vi "Tausand AB1000 Time-Correlated Single Photon Counting Histogram (ContinuousRead) Example.vi"() -> ()   [LabVIEW 2015]
uses:
  <instrlib>/Tausand AB1000/Public/Controls/deviceTypeRing.ctl
  <instrlib>/Tausand AB1000/Public/Controls/channelRing.ctl
  <instrlib>/Tausand AB1000/Public/Controls/settings4ch.ctl
  <instrlib>/Tausand AB1000/Public/Controls/configMultipleCoincRing.ctl
  <vilib>/Utility/error.llb/DialogType.ctl
  <vilib>/Utility/file.llb/Write Delimited Spreadsheet (string).vi
  <vilib>/Analysis/baseanly.llb/Mean (DBL).vi
  <vilib>/Utility/file.llb/Write Delimited Spreadsheet (I64).vi
  <instrlib>/Tausand AB1000/Tausand AB1000.lvlib
  <vilib>/Analysis/NI_AALPro.lvlib
  <vilib>/Analysis/NI_AALBase.lvlib
panel:
  out "read time":timestamp
  out "start time":timestamp
  out "saved headers?":bool
  out "avg data":dbl[][](array[numeric])
  in  "fixed controls":enum32{"Page 1", "Page 2"}(tab)
  in  "Tausand Abacus settings":T1={"sampling"=10, "coincidence_window"=2, "delay_A"=0, "delay_B"=0, "delay_C"=0, "delay_D"=0, "sleep_A"=0, "sleep_B"=0, "sleep_C"=0, "sleep_D"=0, "config_multiple_1"=240} {"config_multiple_1" items=["ABC"=224, "ABD"=208, "ACD"=176, "BCD"=112, "ABCD"=240]; "sleep_D" max=100 step=1; "sleep_C" max=100 step=1; "sleep_B" max=100 step=1; "sleep_A" max=100 step=1; "delay_D" max=100 step=1; "delay_C" max=100 step=1; "delay_B" max=100 step=1; "delay_A" max=100 step=1; "coincidence_window" min=1 max=10000 step=1; "sampling" items=["1ms"=1, "2ms"=2, "3ms"=3, "4ms"=4, "5ms"=5, "6ms"=6, "7ms"=7, "8ms"=8, "9ms"=9, "10ms"=10, "11ms"=11, "12ms"=12, "13ms"=13, "14ms"=14, "15ms"=15, "16ms"=16, "17ms"=17, "18ms"=18, "19ms"=19, "20ms"=20, "21ms"=21, "22ms"=22, "23ms"=23, "24ms"=24, "25ms"=25, "26ms"=26, "27ms"=27, "28ms"=28, "29ms"=29, "30ms"=30, "31ms"=31, "32ms"=32, "33ms"=33, "34ms"=34, "35ms"=35, "36ms"=36, "37ms"=37, "38ms"=38, "39ms"=39, "40ms"=40, "41ms"=41, "42ms"=42, "43ms"=43, "44ms"=44, "45ms"=45, "46ms"=46, "47ms"=47, "48ms"=48, "49ms"=49, "50ms"=50, "51ms"=51, "52ms"=52, "53ms"=53, "54ms"=54, "55ms"=55, "56ms"=56, "57ms"=57, "58ms"=58, "59ms"=59, "60ms"=60, "61ms"=61, "62ms"=62, "63ms"=63, "64ms"=64, "65ms"=65, "66ms"=66, "67ms"=67, "68ms"=68, "69ms"=69, "70ms"=70, "71ms"=71, "72ms"=72, "73ms"=73, "74ms"=74, "75ms"=75, "76ms"=76, "77ms"=77, "78ms"=78, "79ms"=79, "80ms"=80, "81ms"=81, "82ms"=82, "83ms"=83, "84ms"=84, "85ms"=85, "86ms"=86, "87ms"=87, "88ms"=88, "89ms"=89, "90ms"=90, "91ms"=91, "92ms"=92, "93ms"=93, "94ms"=94, "95ms"=95, "96ms"=96, "97ms"=97, "98ms"=98, "99ms"=99, "100ms"=100, "110ms"=110, "120ms"=120, "130ms"=130, "140ms"=140, "150ms"=150, "160ms"=160, "170ms"=170, "180ms"=180, "190ms"=190, "200ms"=200, "210ms"=210, "220ms"=220, "230ms"=230, "240ms"=240, "250ms"=250, "260ms"=260, "270ms"=270, "280ms"=280, "290ms"=290, "300ms"=300, "310ms"=310, "320ms"=320, "330ms"=330, "340ms"=340, "350ms"=350, "360ms"=360, "370ms"=370, "380ms"=380, "390ms"=390, "400ms"=400, "410ms"=410, "420ms"=420, "430ms"=430, "440ms"=440, "450ms"=450, "460ms"=460, "470ms"=470, "480ms"=480, "490ms"=490, "500ms"=500, "510ms"=510, "520ms"=520, "530ms"=530, "540ms"=540, "550ms"=550, "560ms"=560, "570ms"=570, "580ms"=580, "590ms"=590, "600ms"=600, "610ms"=610, "620ms"=620, "630ms"=630, "640ms"=640, "650ms"=650, "660ms"=660, "670ms"=670, "680ms"=680, "690ms"=690, "700ms"=700, "710ms"=710, "720ms"=720, "730ms"=730, "740ms"=740, "750ms"=750, "760ms"=760, "770ms"=770, "780ms"=780, "790ms"=790, "800ms"=800, "810ms"=810, "820ms"=820, "830ms"=830, "840ms"=840, "850ms"=850, "860ms"=860, "870ms"=870, "880ms"=880, "890ms"=890, "900ms"=900, "910ms"=910, "920ms"=920, "930ms"=930, "940ms"=940, "950ms"=950, "960ms"=960, "970ms"=970, "980ms"=980, "990ms"=990, "1,0s"=1000, "1,1s"=1100, "1,2s"=1200, "1,3s"=1300, "1,4s"=1400, "1,5s"=1500, "1,6s"=1600, "1,7s"=1700, "1,8s"=1800, "1,9s"=1900, "2,0s"=2000, "2,1s"=2100, "2,2s"=2200, "2,3s"=2300, "2,4s"=2400, "2,5s"=2500, "2,6s"=2600, "2,7s"=2700, "2,8s"=2800, "2,9s"=2900, "3,0s"=3000, "3,1s"=3100, "3,2s"=3200, "3,3s"=3300, "3,4s"=3400, "3,5s"=3500, "3,6s"=3600, "3,7s"=3700, "3,8s"=3800, "3,9s"=3900, "4,0s"=4000, "4,1s"=4100, "4,2s"=4200, "4,3s"=4300, "4,4s"=4400, "4,5s"=4500, "4,6s"=4600, "4,7s"=4700, "4,8s"=4800, "4,9s"=4900, "5,0s"=5000, "5,1s"=5100, "5,2s"=5200, "5,3s"=5300, "5,4s"=5400, "5,5s"=5500, "5,6s"=5600, "5,7s"=5700, "5,8s"=5800, "5,9s"=5900, "6,0s"=6000, "6,1s"=6100, "6,2s"=6200, "6,3s"=6300, "6,4s"=6400, "6,5s"=6500, "6,6s"=6600, "6,7s"=6700, "6,8s"=6800, "6,9s"=6900, "7,0s"=7000, "7,1s"=7100, "7,2s"=7200, "7,3s"=7300, "7,4s"=7400, "7,5s"=7500, "7,6s"=7600, "7,7s"=7700, "7,8s"=7800, "7,9s"=7900, "8,0s"=8000, "8,1s"=8100, "8,2s"=8200, "8,3s"=8300, "8,4s"=8400, "8,5s"=8500, "8,6s"=8600, "8,7s"=8700, "8,8s"=8800, "8,9s"=8900, "9,0s"=9000, "9,1s"=9100, "9,2s"=9200, "9,3s"=9300, "9,4s"=9400, "9,5s"=9500, "9,6s"=9600, "9,7s"=9700, "9,8s"=9800, "9,9s"=9900, "10s"=10000, "11s"=11000, "12s"=12000, "13s"=13000, "14s"=14000, "15s"=15000, "16s"=16000, "17s"=17000, "18s"=18000, "19s"=19000, "20s"=20000, "21s"=21000, "22s"=22000, "23s"=23000, "24s"=24000, "25s"=25000, "26s"=26000, "27s"=27000, "28s"=28000, "29s"=29000, "30s"=30000, "31s"=31000, "32s"=32000, "33s"=33000, "34s"=34000, "35s"=35000, "36s"=36000, "37s"=37000, "38s"=38000, "39s"=39000, "40s"=40000, "41s"=41000, "42s"=42000, "43s"=43000, "44s"=44000, "45s"=45000, "46s"=46000, "47s"=47000, "48s"=48000, "49s"=49000, "50s"=50000, "51s"=51000, "52s"=52000, "53s"=53000, "54s"=54000, "55s"=55000, "56s"=56000, "57s"=57000, "58s"=58000, "59s"=59000, "60s"=60000, "61s"=61000, "62s"=62000, "63s"=63000, "64s"=64000, "65s"=65000, "66s"=66000, "67s"=67000, "68s"=68000, "69s"=69000, "70s"=70000, "71s"=71000, "72s"=72000, "73s"=73000, "74s"=74000, "75s"=75000, "76s"=76000, "77s"=77000, "78s"=78000, "79s"=79000, "80s"=80000, "81s"=81000, "82s"=82000, "83s"=83000, "84s"=84000, "85s"=85000, "86s"=86000, "87s"=87000, "88s"=88000, "89s"=89000, "90s"=90000, "91s"=91000, "92s"=92000, "93s"=93000, "94s"=94000, "95s"=95000, "96s"=96000, "97s"=97000, "98s"=98000, "99s"=99000, "100s"=100000, "110s"=110000, "120s"=120000, "130s"=130000, "140s"=140000, "150s"=150000, "160s"=160000, "170s"=170000, "180s"=180000, "190s"=190000, "200s"=200000, "210s"=210000, "220s"=220000, "230s"=230000, "240s"=240000, "250s"=250000, "260s"=260000, "270s"=270000, "280s"=280000, "290s"=290000, "300s"=300000, "310s"=310000, "320s"=320000, "330s"=330000, "340s"=340000, "350s"=350000, "360s"=360000, "370s"=370000, "380s"=380000, "390s"=390000, "400s"=400000, "410s"=410000, "420s"=420000, "430s"=430000, "440s"=440000, "450s"=450000, "460s"=460000, "470s"=470000, "480s"=480000, "490s"=490000, "500s"=500000, "510s"=510000, "520s"=520000, "530s"=530000, "540s"=540000, "550s"=550000, "560s"=560000, "570s"=570000, "580s"=580000, "590s"=590000, "600s"=600000, "610s"=610000, "620s"=620000, "630s"=630000, "640s"=640000, "650s"=650000, "660s"=660000, "670s"=670000, "680s"=680000, "690s"=690000, "700s"=700000, "710s"=710000, "720s"=720000, "730s"=730000, "740s"=740000, "750s"=750000, "760s"=760000, "770s"=770000, "780s"=780000, "790s"=790000, "800s"=800000, "810s"=810000, "820s"=820000, "830s"=830000, "840s"=840000, "850s"=850000, "860s"=860000, "870s"=870000, "880s"=880000, "890s"=890000, "900s"=900000, "910s"=910000, "920s"=920000, "930s"=930000, "940s"=940000, "950s"=950000, "960s"=960000, "970s"=970000, "980s"=980000, "990s"=990000, "1000s"=1000000]}
  in  "device type":T3 items=["any"=0, "AB1002"=1002, "AB1004"=1004, "AB1502"=1502, "AB1504"=1504, "AB2002"=2002, "AB2004"=2004, "AB2502"=2502, "AB2504"=2504]
  in  "VISA resource name":refnum<visa-resource-name>
  in  "first ch":T4=1 caption="first channel" items=["none", "A", "B", "C", "D", "E", "F", "G", "H"]
  in  "second ch":T4=2 caption="second channel" items=["none", "A", "B", "C", "D", "E", "F", "G", "H"]
  in  "resolution":u32(ring)=2 items=["2ns"=2, "10ns"=10, "100ns"=100]
  in  "numbins":i32=50
  out "averaged histograms":i32
  out "avg TCSPC":dbl[](array[numeric])
  out "avg TCSPC hist":cluster{u32[], u32[]}(graph) caption="averaged TCSPC histogram"
  out "avg coinc graph":cluster{u32[], u32[]}(graph) caption="averaged cumulative coincidences"
  out "avg coinc":dbl[](array[numeric])
  out "coinc matrix":u32[][](array[numeric])
  in  "Clear Button":bool
  in  "stop":bool
  out "progress":dbl(slide) scale=0.0..1.0
  in  "Save to file?":bool
  in  "Path":path
  out "data":u32[][](array[numeric])
  out "TCSPC array":u32[](array[numeric])
  out "coinc graph":cluster{u32[], u32[]}(graph) caption="cumulative coincidences"
  out "TCSPC hist":cluster{u32[], u32[]}(graph) caption="TCSPC histogram"
  out "coinc array":u32[](array[numeric])
  out "coinc value":u32
  out "checksum ok?":bool
  out "cw array":u32[](array[numeric])
  # "Overview: example of building a time-correlated single photon counting (TCSPC) histogram using a Tausand Abacus AB1502, AB1504, AB2502 or AB2504 device. This example builds the histogram continously and saves each TCSPC data in a file.\nInstructions:\n1. Before running the VI:\n*Select the VISA port AND the Device type\n*Select the start/stop input channels\n*Select histogram settings: resolution (2ns,10ns, or 100ns), and number of bins (máx. 50 for 2ns, máx. 100 otherwise).\n*Set the sampling time per bin. Recommended value: 10ms.\n*Set delays and sleep times, if required.\n2. Run the VI\n3. TCSPC data will be saved, if selected.\n4. Press 'STOP' to stop the VI."
  # "October 2023"
  # "máx: 100 (50 for 2ns)"
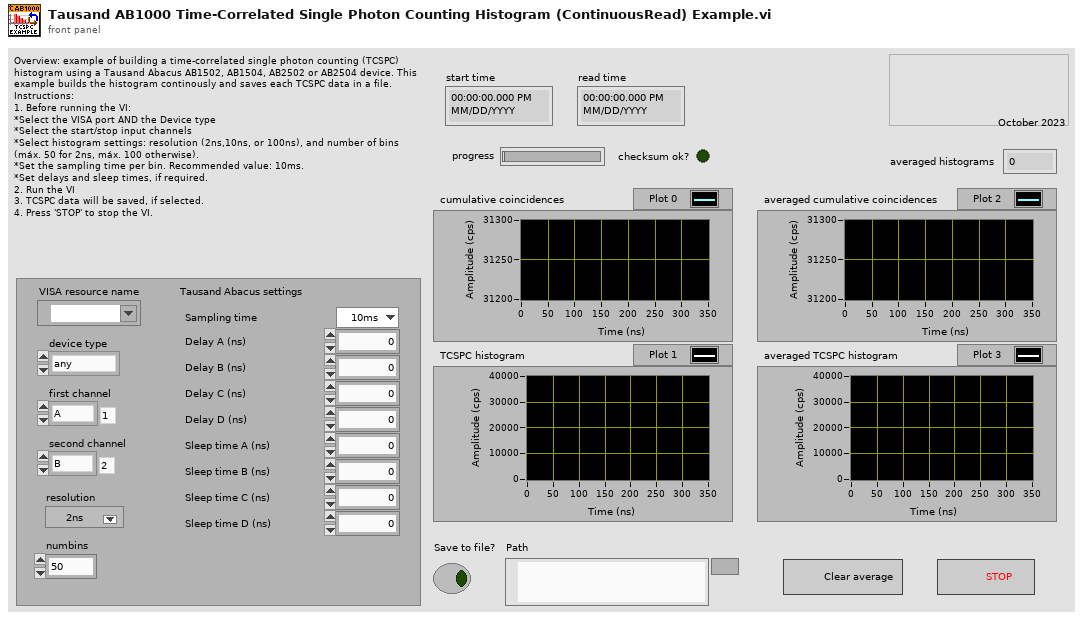
[diagram p1: front panel]
types:
  T1 = typedef "Tausand AB1000.lvlib/settings4ch.ctl" = cluster{"sampling":u32, "coincidence_window":u32, "delay_A":u32, "delay_B":u32, "delay_C":u32, "delay_D":u32, "sleep_A":u32, "sleep_B":u32, "sleep_C":u32, "sleep_D":u32, "config_multiple_1":T2}
  T2 = typedef "Tausand AB1000.lvlib/configMultipleCoincRing.ctl" = u16
  T3 = typedef "Tausand AB1000.lvlib/deviceTypeRing.ctl" = u16
  T4 = typedef "Tausand AB1000.lvlib/channelRing.ctl" = u8
  T5 = enum8{"Enabled", "Disabled", "Disabled and Grayed Out"}
  T6 = typedef "DialogType.ctl" = u16
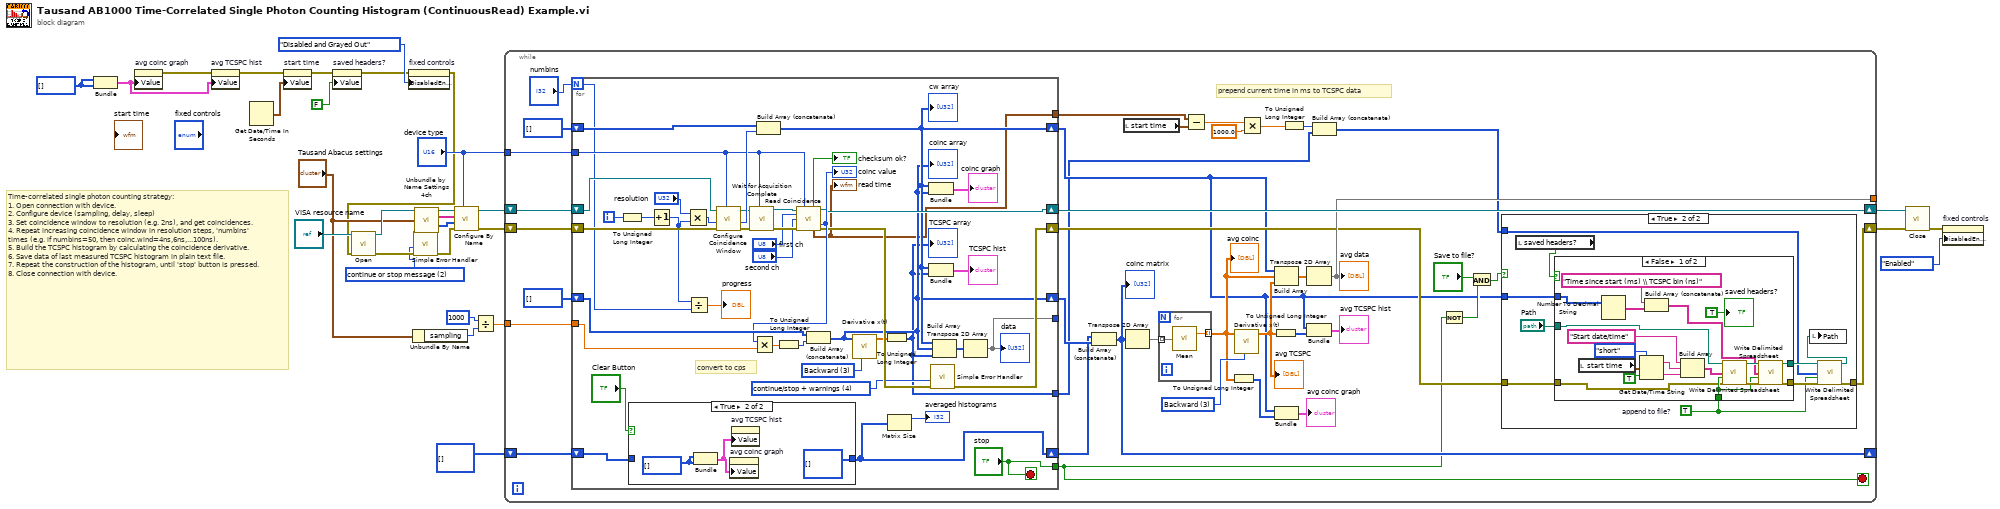
[diagram p0: block diagram]
diagram:
  w4 = u32[] []
  w14 = T6 2 items=["no dialog", "OK message", "continue or stop message", "OK message + warnings", "continue/stop + warnings"] ("type of dialog (OK msg:1)")
  # "Time-correlated single photon counting strategy:\n1. Open connection with device.\n2. Configure device (sampling, delay, sleep)\n3. Set coincidence window to resolution (e.g. 2ns), and get coincidences.\n4. Repeat increasing coincidence window in resolution steps, 'numbins' times (e.g. if numbins=50, then coinc.wind=4ns,6ns,...100ns).\n5. Build the TCSPC histogram by calculating the coincidence derivative.\n6. Save data of last measured TCSPC histogram in plain text file.\n7. Repeat the construction of the histogram, until 'stop' button is pressed. \n8. Close connection with device."
  n1 = Bundle(w4, w4) -> (w3:cluster{u32[], u32[]})  [unwired: 1 in]
  n2 = property on="avg coinc graph" class="XYGraph (strict)"("Value"=w3) -> (error out=w1:errorcluster)  [unwired: 2 in, 1 out]
  n3 = property on="avg TCSPC hist" class="XYGraph (strict)"(error in=w1, "Value"=w3) -> (error out=w2:errorcluster)  [unwired: 1 in, 1 out]
  n4 = Get Date/Time In Seconds() -> (seconds since 1Jan1904=w5:timestamp)
  n5 = property on="start time" class="AbsTime (strict)"(error in=w2, "Value"=w5) -> (error out=w6:errorcluster)  [unwired: 1 in, 1 out]
  n6 = property on="saved headers?" class="Bool (strict)"(error in=w6, "Value"=FALSE ("saved headers?")) -> (error out=w7:errorcluster)  [unwired: 1 in, 1 out]
  n7 = property on="fixed controls" class="TabCtl (strict)"(error in=w7, "DisabledEnum"=T5."Disabled and Grayed Out" ("Disabled")) -> (error out=w11:errorcluster)  [unwired: 1 in, 1 out]
  n8 = call <instrlib>:"Open.vi"("error in (no error)"=w11, "VISA resource name"="VISA resource name") -> ("error out"=w16:errorcluster, "VISA resource name out"=w27:refnum<visa-resource-name>)  [unwired: 8 in]
  n9 = Unbundle By Name("Tausand Abacus settings") -> ("sampling"=w19:u32)
  n10 = call <vilib>:"Simple Error Handler.vi"("type of dialog (OK msg:1)"=w14, "error in (no error)"=w16) -> ("error out"=w15:errorcluster)  [unwired: 3 in, 4 out]
  n11 = call <instrlib>:"Unbundle by Name Settings 4ch.vi"("input cluster settings 4ch"="Tausand Abacus settings") -> ("names"=w24:string[], "values"=w23:u32[])  [unwired: 13 in]
  n12 = call <instrlib>:"Configure By Name.vi"("device type"="device type", "error in (no error)"=w15, "values"=w23, "labels"=w24, "VISA Refnum in"=w27) -> ("error out"=w29:errorcluster, "VISA Refnum out"=w26:refnum<visa-resource-name>)  [unwired: 5 in]
  n13 = Divide(x=u32 1000, y=w19) -> (x/y=w17:dbl)
  n14 = while {
    tunnel: "device type" -> [w63]
    tunnel: w17 -> [w59]
    shift-right: [w43] -> w28
    shift-left: w29 -> [w66]
    shift-right: [w64] -> w25
    shift-left: w26 -> [w65]
    shift-right: [w57] -> _
    shift-left: u32[][] [] -> [w49]
    tunnel: [w46] -> _
    stop <- w39 stop-if-true
    w55 = u16 3 items=["2nd Order Central", "4th Order Central", "Forward", "Backward"] ("method")
    # "prepend current time in ms to TCSPC data"
    n15 = for {
      N: "numbins" -> [w107]
      shift-right: [w115] -> w44
      shift-left: w66 -> [w141]
      shift-right: [w117] -> w64
      shift-left: w65 -> [w140]
      tunnel: w63 -> [w118]
      shift-right: [w113] -> w35
      shift-left: u32[] [] -> [w123]
      shift-right: [w112] -> w58
      shift-left: i32[] [] -> [w127]
      tunnel: w59 -> [w121]
      tunnel: [w110] -> _
      tunnel: ["stop"] -> w39
      shift-right: [w102] -> w50
      shift-left: w49 -> [w103]
      tunnel: [w100] -> w34
      tunnel: [w99] -> w30
      i -> [w137]
      stop <- "stop" stop-if-true
      w114 = T6 4 items=["no dialog", "OK message", "continue or stop message", "OK message + warnings", "continue/stop + warnings"] ("type of dialog (OK msg:1)")
      w126 = u16 3 items=["2nd Order Central", "4th Order Central", "Forward", "Backward"] ("method")
      # "convert to cps"
      n16 = To Unsigned Long Integer(number=w137) -> (unsigned 32bit integer=w136:u32)
      n17 = case shown="True" "Clear Button" {
        tunnel: [w142 u32[][] [] ("t")] -> w102
        tunnel: w103 -> [w142 _]
        frame False {
        }
        frame True {
          w144 = u32[] []
          n18 = Bundle(w144, w144) -> (w143:cluster{u32[], u32[]})  [unwired: 1 in]
          n19 = property on="avg coinc graph" class="XYGraph (strict)"("Value"=w143) -> ()  [unwired: 2 in, 2 out]
          n20 = property on="avg TCSPC hist" class="XYGraph (strict)"("Value"=w143) -> ()  [unwired: 2 in, 2 out]
        }
      }
      n21 = Increment(x=w136) -> (x+1=w108:u32)
      n22 = Multiply(x="resolution", y=w108) -> (x*y=w139:u32)
      n23 = Divide(x=w108, y=w107) -> (x/y=→"progress":dbl)
      n24 = call <instrlib>:"Configure Coincidence Window.vi"("device type"=w118, "error in (no error)"=w141, "value ns (10ns)"=w139, "VISA Refnum in"=w140) -> ("error out"=w134:errorcluster, "value ns out"=w135:u32, "VISA Refnum out"=w128:refnum<visa-resource-name>)  [unwired: 5 in]
      n25 = call <instrlib>:"Wait for Acquisition Complete.vi"("device type"=w118, "error in (no error)"=w134, "VISA resource name"=w128) -> ("error out"=w133:errorcluster, "VISA resource name out"=w132:refnum<visa-resource-name>)  [unwired: 7 in]
      n26 = Build Array (concatenate)(w123, w135) -> (w113:u32[])
      "cw array" <- w113
      n27 = call <instrlib>:"Read Coincidence.vi"("VISA Refnum in"=w132, "device type"=w118, "first ch"="first ch", "second ch"="second ch", "error in (no error)"=w133) -> ("checksum ok?"=→"checksum ok?":bool, "VISA Refnum out"=w117:refnum<visa-resource-name>, "value"=w122:u32, "read time"=w99:timestamp, "error out"=w116:errorcluster)  [unwired: 5 in, 1 out]
      "coinc value" <- w122
      "read time" <- w99
      n28 = Multiply(x=w122, y=w121) -> (x*y=w120:dbl)
      n29 = To Unsigned Long Integer(number=w120) -> (unsigned 32bit integer=w119:u32)
      n30 = Build Array (concatenate)(w127, w119) -> (w112:u32[])
      "coinc array" <- w112
      n31 = call <vilib>:"Derivative x(t).vi"("method"=w126, "X"=w112) -> ("dX/dt"=w109:dbl[])  [unwired: 8 in, 1 out]
      n32 = To Unsigned Long Integer(number=w109) -> (unsigned 32bit integer=w100:u32[])
      "TCSPC array" <- w100
      n33 = Matrix Size(0:w102) -> (1:→"averaged histograms":i32)  [unwired: 1 out]
      n34 = Bundle(w113, w112) -> (→"coinc graph":cluster{u32[], u32[]})  [unwired: 1 in]
      n35 = Bundle(w113, w100) -> (→"TCSPC hist":cluster{u32[], u32[]})  [unwired: 1 in]
      n36 = call <vilib>:"Simple Error Handler.vi"("type of dialog (OK msg:1)"=w114, "error in (no error)"=w116) -> ("error out"=w115:errorcluster)  [unwired: 3 in, 4 out]
      n37 = Build Array(w113, w112, w100) -> (w111:u32[][])
      n38 = Transpose 2D Array(2D array=w111) -> (transposed array=w110:u32[][])
      "data" <- w110
    }
    n39 = Build Array (concatenate)(w50, w58) -> (w57:u32[][])
    "coinc matrix" <- w57
    n40 = local read "start time"() -> (w33:timestamp)
    n41 = Transpose 2D Array(2D array=w57) -> (transposed array=w51:u32[][])
    n42 = for {
      tunnel: w51 -> [w147] mode=indexing
      tunnel: [w146] -> w47 mode=indexing
      n43 = call-poly <vilib>:"Mean.vi"("X"=w147) -> ("mean"=w146:dbl)  [unwired: 1 out]
    }
    "avg coinc" <- w47
    n44 = Subtract(x=w30, y=w33) -> (x-y=w32:dbl)
    n45 = To Unsigned Long Integer(number=w47) -> (unsigned 32bit integer=w52:u32[])
    n46 = call <vilib>:"Derivative x(t).vi"("method"=w55, "X"=w47) -> ("dX/dt"=w45:dbl[])  [unwired: 8 in, 1 out]
    "avg TCSPC" <- w45
    n47 = Multiply(x=w32, y=1000.0) -> (x*y=w38:dbl)
    n48 = To Unsigned Long Integer(number=w45) -> (unsigned 32bit integer=w53:u32[])
    n49 = Build Array(w35, w47, w45) -> (w48:dbl[][])
    n50 = Bundle(w35, w52) -> (→"avg coinc graph":cluster{u32[], u32[]})  [unwired: 1 in]
    n51 = To Unsigned Long Integer(number=w38) -> (unsigned 32bit integer=w37:u32)
    n52 = Transpose 2D Array(2D array=w48) -> (transposed array=w46:dbl[][])
    "avg data" <- w46
    n53 = Bundle(w35, w53) -> (→"avg TCSPC hist":cluster{u32[], u32[]})  [unwired: 1 in]
    n54 = Build Array (concatenate)(w37, w34) -> (w36:u32[])
    n55 = Not(x=w39) -> (.not. x?=w40:bool)
    n56 = And(x="Save to file?", y=w40) -> (x .and. y?=w41:bool)
    n57 = case shown="True" w41 {
      tunnel: w36 -> [_ w72]
      tunnel: w44 -> [w67 w74]
      tunnel: [w67 w73] -> w43
      tunnel: w35 -> [_ w68]
      frame False {
      }
      frame True {
        w75 = TRUE  # append to file?
        n58 = local read "saved headers?"() -> (w71:bool)
        n59 = case shown="False" w71 {
          tunnel: [w96 w98] -> w77
          tunnel: [w95 w97] -> w76
          tunnel: w75 -> [w88 _]
          tunnel: w74 -> [w87 w97]
          tunnel: "Path" -> [w86 w98]
          tunnel: w68 -> [w79 _]
          frame False {
            n60 = local read "start time"() -> (w82:timestamp)
            n61 = Number To Decimal String(number=w79) -> (decimal integer string=w80:string[])  [unwired: 1 in]
            n62 = Get Date/Time String(date format (0)=enum16{"short", "long", "abbreviated"}."short", seconds (now)=w82, want seconds? (F)=TRUE) -> (date string=w92:string, time string=w93:string)
            n63 = Build Array (concatenate)("Time since start (ms) \\ TCSPC bin (ns)", w80) -> (w78:string[])
            n64 = Build Array("Start date/time", w92, w93) -> (w89:string[])
            n65 = call-poly <vilib>:"Write Delimited Spreadsheet.vi"("file path (dialog if empty)"=w86, "1D data"=w89, "append to file? (F)"=w88, "error in (no error)"=w87) -> ("new file path (Not A Path if cancelled)"=w85:path, "error out"=w94:errorcluster)  [unwired: 10 in]
            n66 = call-poly <vilib>:"Write Delimited Spreadsheet.vi"("file path (dialog if empty)"=w85, "1D data"=w78, "append to file? (F)"=w88, "error in (no error)"=w94) -> ("new file path (Not A Path if cancelled)"=w96:path, "error out"=w95:errorcluster)  [unwired: 10 in]
            "saved headers?" <- TRUE ("saved headers?")
          }
          frame True {
          }
        }
        n67 = call-poly <vilib>:"Write Delimited Spreadsheet.vi"("file path (dialog if empty)"=w77, "1D data"=w72, "append to file? (F)"=w75, "error in (no error)"=w76) -> ("new file path (Not A Path if cancelled)"=w69:path, "error out"=w73:errorcluster)  [unwired: 10 in]
        n68 = local write "Path"(w69) -> ()
      }
    }
  }
  n69 = call <instrlib>:"Close.vi"("error in (no error)"=w28, "VISA resource name"=w25) -> ("error out"=w9:errorcluster)  [unwired: 9 in]
  n70 = property on="fixed controls" class="TabCtl (strict)"(error in=w9, "DisabledEnum"=T5."Enabled" ("Disabled")) -> ()  [unwired: 1 in, 2 out]
